vi "Set_DwellTime.vi"(11 "Tau":i32=2) -> (3 "Next Dwell":i32)   [LabVIEW 2020]
uses:
  <vilib>/gmath/statdist.llb/Exp Random.vi
  <vilib>/gmath/NI_Gmath.lvlib
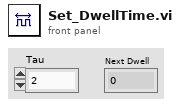
[diagram p1: front panel]
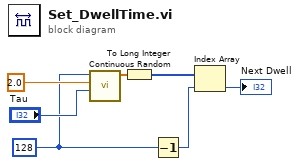
[diagram p0: block diagram]
diagram:
  w3 = 128 ("Trial")
  n1 = call-poly <vilib>:"Continuous Random.vi"("b"="Tau", "a"=2.0, "samples"=w3) -> ("exp random data"=w5:dbl[])  [unwired: 7 in, 1 out]
  n2 = To Long Integer(number=w5) -> (32bit integer=w4:i32[])
  n3 = Decrement(x=w3) -> (x-1=w2:i32)
  n4 = Index Array(array=w4, index=w2) -> (element=→"Next Dwell":i32)
